vi "Actor Core.vi"(8 "error in":errorcluster, 11 "Special Monitor in":refnum<class "Special Monitor.lvclass">) -> (0 "error out":errorcluster, 3 "Actor out":refnum<class "Actor.lvclass">)   [LabVIEW 2017, in "Special Monitor.lvclass"]
doc: "(<B>Filename</B>: Actor Framework.lvlib:Actor.lvclass:Actor Core.vi)\n\nReceives messages to the actor, reacts to them, and initiates any error handling that may shut the actor down.\n\nDescendant classes may override this VI to append parallel tasks for the actor to complete while it handles messages. Overrides use the Call Parent Method node."
uses:
  Special Monitor.lvclass
  <vilib>/ActorFramework/Actor/Actor.lvclass
  <vilib>/ActorFramework/Message Enqueuer/Message Enqueuer.lvclass
  monitored-actor-core/Source/Monitor Data/Monitor Data.lvclass
  Special Monitor.lvclass/Special Monitor.ctl
  <vilib>/ActorFramework/Message Enqueuer/Message Enqueuer.lvclass/Message Enqueuer.ctl
  <vilib>/ActorFramework/Message Enqueuer/Enqueue.vi
  <vilib>/ActorFramework/Stop Msg/Stop Msg.lvclass
  C:/Program Files (x86)/National Instruments/LabVIEW 2017/vi.lib/ActorFramework/Message/Message.lvclass
  <vilib>/ActorFramework/Message Priority Queue/Priority Enqueue.vi
  monitored-actor-core/Source/Actor Monitor/Actor Monitor/Actor Monitor.lvclass
panel:
  in  "Stop All":bool
  out "Actor Count":i32
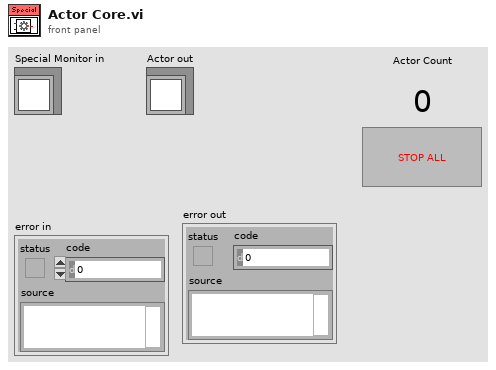
[diagram p1: front panel]
types:
  T1 = cluster{"Monitor Data":refnum<class "Monitor Data.lvclass">, "Changed Actor Q":refnum<class "Message Enqueuer.lvclass">}
  T2 = enum32{"Invalid", "Standard", "Closed", "Hidden", "Minimized", "Maximized"}
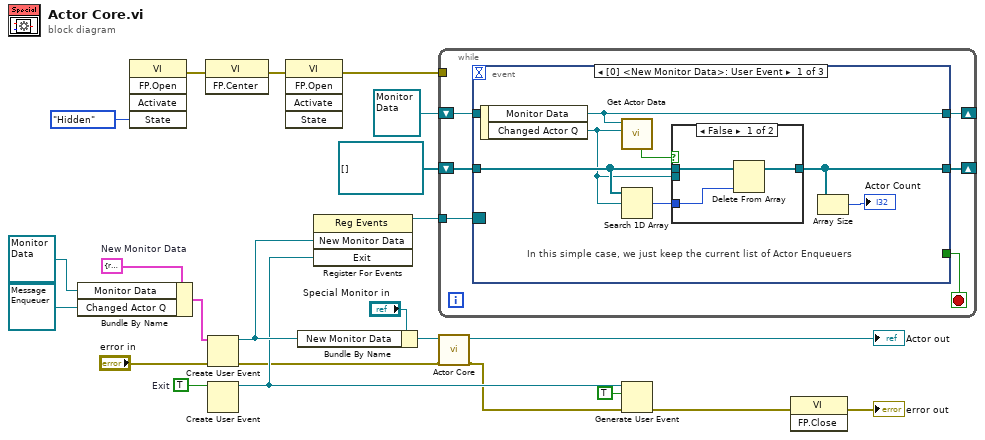
[diagram p0: block diagram]
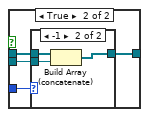
[diagram p2: hidden frame]
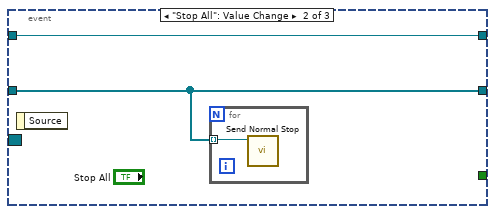
[diagram p4: hidden frame]
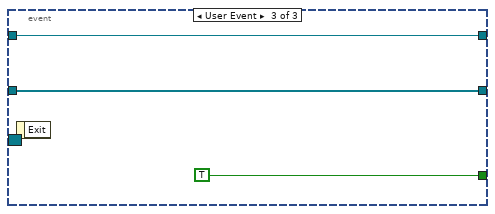
[diagram p5: hidden frame]
diagram:
  w19 = T1 {"Monitor Data"=refnum, "Changed Actor Q"=refnum}  # New Monitor Data
  w14 = TRUE  # Exit
  n1 = Bundle By Name(cluster=w19, "Monitor Data"=refnum<class "Monitor Data.lvclass"> refnum, "Changed Actor Q"=refnum<class "Message Enqueuer.lvclass"> refnum) -> (w18:T1)
  n2 = invoke class="VI" method="FP.Open"("State"=T2."Hidden") -> (error out=w8:errorcluster)  [unwired: 4 in, 4 out]
  n3 = invoke class="VI" method="FP.Center"(error in=w8) -> (error out=w9:errorcluster)  [unwired: 2 in, 2 out]
  n4 = Create User Event(user event datatype=w18, error in="error in") -> (user event=w17:refnum<user-event>, error out=w2:errorcluster)
  n5 = Create User Event(user event datatype=w14) -> (user event=w12:refnum<user-event>)  [unwired: 1 in, 1 out]
  n6 = invoke class="VI" method="FP.Open"(error in=w9) -> (error out=w7:errorcluster)  [unwired: 4 in, 4 out]
  n7 = Bundle By Name(cluster="Special Monitor in", "New Monitor Data"=w17) -> (w3:refnum<class "Special Monitor.lvclass">)
  n8 = register-events(w17, w12) -> (reference out=w22:refnum<event-registration>)  [unwired: 2 in, 1 out]
  n9 = while {
    tunnel: w22 -> [w29]
    shift-right: [w25] -> _
    shift-left: refnum<class "Message Enqueuer.lvclass">[] [] -> [w26]
    shift-right: [w28] -> _
    shift-left: refnum<class "Monitor Data.lvclass"> refnum ("Monitor Data") -> [w27]
    tunnel: w7 -> [_]
    stop <- w24 stop-if-true
    n10 = event shown="[0] <New Monitor Data>: User Event" {
      selector: w29 -> [_ _ _]
      dyn-events: _ -> [_ _ _]
      timeout: _ -> [_ _ _]
      tunnel: [w34 w49 w52] -> w28
      tunnel: w27 -> [_ w49 w52]
      tunnel: w26 -> [w35 w48 w53]
      tunnel: [w31 w48 w53] -> w25
      tunnel: [_ _ TRUE] -> w24
      event User Event {
        # "In this simple case, we just keep the current list of Actor Enqueuers"
        n11 = event-data() -> ("Monitor Data"=w34:refnum<class "Monitor Data.lvclass">, "Changed Actor Q"=w33:refnum<class "Message Enqueuer.lvclass">)  [unwired: 1 in]
        n12 = call "Get Actor Data.vi"("Actor's Self Q"=w33, "Monitor Data in"=w34) -> ("Found?"=w32:bool)  [unwired: 6 in, 3 out]
        n13 = Search 1D Array(1D array=w35, element=w33) -> (index of element=w36:i32)  [unwired: 1 in]
        n14 = case shown="False" w32 {
          tunnel: w36 -> [w38 w43]
          tunnel: w35 -> [w39 w42]
          tunnel: [w37 w41] -> w31
          tunnel: w33 -> [_ w40]
          frame False {
            n15 = Delete From Array(array=w39, index=w38) -> (array with subset deleted=w37:refnum<class "Message Enqueuer.lvclass">[])  [unwired: 1 in, 1 out]
          }
          frame True {
            n16 = case shown="-1" w43 {
              tunnel: [w44 w47] -> w41
              tunnel: w42 -> [w44 w46]
              tunnel: w40 -> [_ w45]
              frame Default {
              }
              frame -1 {
                n17 = Build Array (concatenate)(w46, w45) -> (w47:refnum<class "Message Enqueuer.lvclass">[])
              }
            }
          }
        }
        n18 = Array Size(array=w31) -> (size(s)=→"Actor Count":i32)
      }
      event "Stop All": Value Change {
        n19 = event-data() -> ()  [unwired: 1 in, 1 out]
        n20 = for {
          tunnel: w48 -> [w50] mode=indexing
          n21 = call <vilib>:"Send Normal Stop.vi"("Message Enqueuer"=w50) -> ()  [unwired: 10 in, 1 out]
        }
      }
      event User Event {
        n22 = event-data() -> ()  [unwired: 1 in, 1 out]
      }
    }
  }
  n23 = call-parent "Actor Core.vi"("error in"=w2, "Actor in"=w3) -> ("error out"=w1:errorcluster, "Actor out"=→"Actor out":refnum<class "Actor.lvclass">)  [unwired: 8 in]
  n24 = Generate User Event(user event=w12, event data cluster=TRUE ("event data"), error in=w1) -> (error out=w11:errorcluster)  [unwired: 1 in, 1 out]
  n25 = invoke class="VI" method="FP.Close"(error in=w11) -> (error out=→"error out":errorcluster)  [unwired: 2 in, 2 out]
